vi "Handle Message.vi"(0 "ICanComunicate In":refnum<class "Process.lvclass">, 7 "Message In":T1, 11 "Error In":errorcluster) -> (4 "ICanComunicate Out":refnum<class "Process.lvclass">, 6 "CMD Out":string, 8 "Message Out":T1, 15 "Error Out":errorcluster)   [LabVIEW 2023, in "Process.lvclass"]
uses:
  Process.lvclass
  Interfaces/ICanCommunicate/Message.ctl
  Process.lvclass/Process.ctl
  Interfaces/ICanCommunicate/ICanCommunicate.lvclass
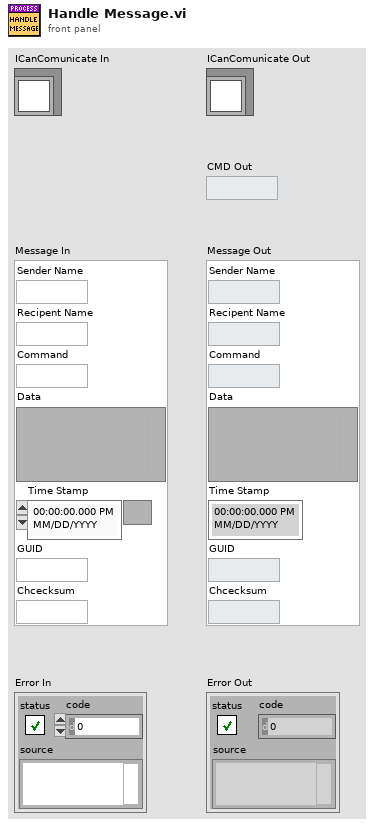
[diagram p1: front panel]
types:
  T1 = typedef "ICanCommunicate.lvclass/Message.ctl" = cluster{"Sender Name":string, "Recipent Name":string, "Command":string, "Data":variant, "Time Stamp":timestamp, "GUID":string, "Chcecksum":string}
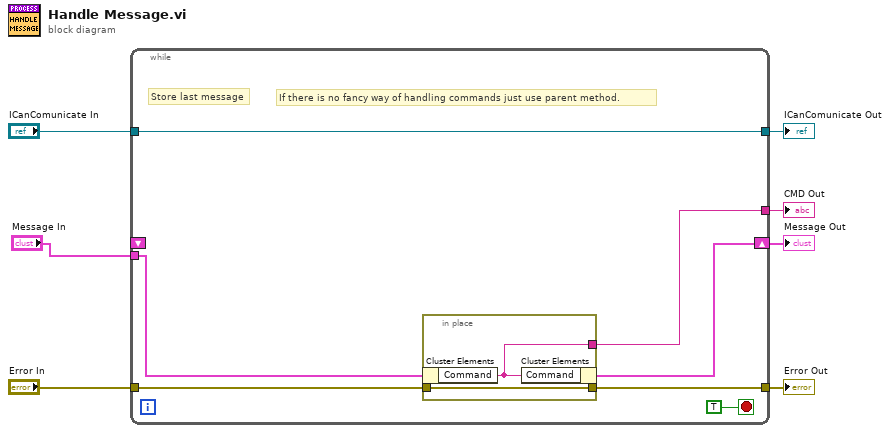
[diagram p0: block diagram]
diagram:
  n1 = while {
    shift-right: [w9] -> w3
    shift-left: _ -> [_]
    tunnel: "Error In" -> [w13]
    tunnel: [w8] -> w6
    tunnel: "ICanComunicate In" -> [w11]
    tunnel: [w11] -> w4
    tunnel: "Message In" -> [w12]
    tunnel: [w10] -> w1
    stop <- TRUE stop-if-true
    # "If there is no fancy way of handling commands just use parent method."
    # "Store last message"
    n2 = in-place {
      in-place-border: [w15] -> w10
      in-place-border: [w16] -> w8
      in-place-border: w13 -> [w16]
      n3 = in-place-cluster #1(w12) -> ("Command"=w15:string)
      n4 = in-place-cluster #1("Command"=w15) -> (w9:T1)
    }
  }
  "Error Out" <- w6
  "ICanComunicate Out" <- w4
  "Message Out" <- w3
  "CMD Out" <- w1
